vi "11d-async.vi"() -> ()   [LabVIEW 2018, in "LV2Julia_examples.lvlib"]
uses:
  LV2Julia_examples.lvlib
  LV2Julia_core/VIs/Server or client state.ctl
  LV2Julia_core/VIs/detailed error info.ctl
  LV2Julia_core/VIs/StackFrame.ctl
  LV2Julia_core/VIs/Commands.ctl
  be4745b6-8471-45fc-b8a0-8968ce92ea4b.vi
  be4745b6-8471-45fc-b8a0-8968ce92ea4b.vi/01ce1741-ea78-47f8-98ed-e79163fb1a9b.vi
  be4745b6-8471-45fc-b8a0-8968ce92ea4b.vi/01ce1741-ea78-47f8-98ed-e79163fb1a9b.vi/cc3cf2af-bc3b-4fb6-855b-7562c4d0bfeb.vi
  be4745b6-8471-45fc-b8a0-8968ce92ea4b.vi/01ce1741-ea78-47f8-98ed-e79163fb1a9b.vi/c77cecd8-10de-4d46-bc1c-57302a887fda.vi
  be4745b6-8471-45fc-b8a0-8968ce92ea4b.vi/01ce1741-ea78-47f8-98ed-e79163fb1a9b.vi/2cafb1dd-d397-4b79-911a-06d102936120.vi
  LV2Julia_core/VIs/jl-scripts path.vi
  LV2Julia_core/VIs/check ID validity.vi
  LV2Julia_core/VIs/bindata_descr to JSON.vi
  LV2Julia_core/VIs/check cluster field names.vi
  LV2Julia_core/VIs/concat JSON.vi
  LV2Julia_core/VIs/build request.vi
  LV2Julia_core/VIs/Parse server response.vi
  LV2Julia_core/VIs/log jl exceptions.vi
  LV2Julia_core/LV2Julia_core.lvlib
panel:
  in  "Timeout (s)":dbl=-1.0
  out "Boolean":bool
  out "notification":bool
  in  "stop polling":bool
  out "stopping":bool
  out "done":bool
  in  "summands":cluster{"x":dbl, "y":dbl}={"x"=2.0, "y"=2.0}
  in  "next":bool
  out "x+y":dbl=nan
  out "detailed error info":T1
  out "current error":errorcluster
  out "final error":errorcluster
  out "short err code":u8
  in  "stop":bool
  out "ZMQ timeout":bool
  out "Julia script file path":path
  out "temporary script path":path
  out "Jl Server state":T3
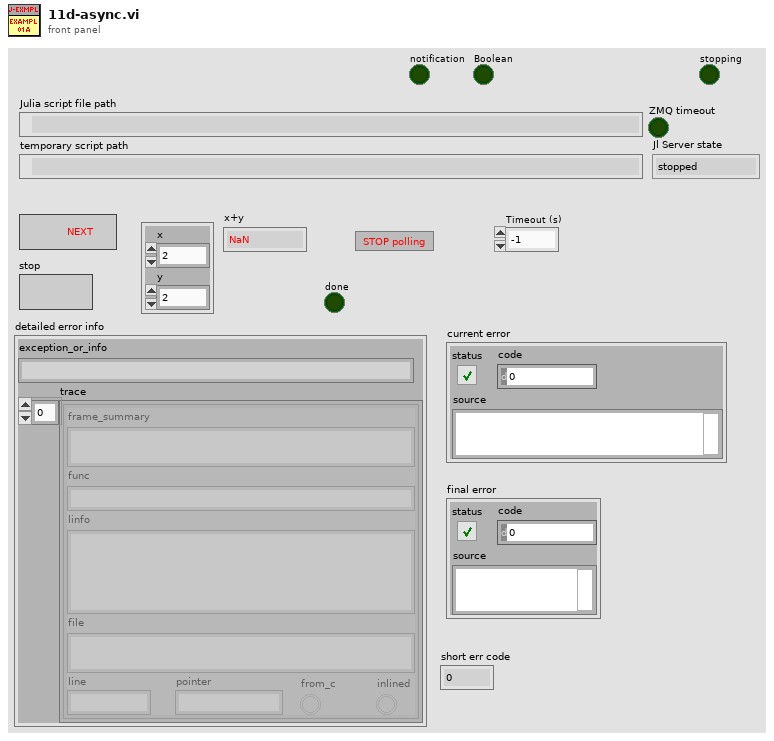
[diagram p1: front panel]
types:
  T1 = typedef "LV2Julia_core.lvlib/detailed error info.ctl" = cluster{"exception_or_info":string, "trace":T2[]}
  T2 = typedef "LV2Julia_core.lvlib/StackFrame.ctl" = cluster{"frame_summary":string, "func":string, "linfo":string, "file":string, "line":i32, "pointer":u64, "from_c":bool, "inlined":bool}
  T3 = typedef "LV2Julia_core.lvlib/Server or client state.ctl" = enum16{"stopped", "running", "unknown"}
  T4 = typedef "LV2Julia_core.lvlib/Commands.ctl" = enum16{"Start Jl-server & Init LV-client", "Send request & Get response ", "Stop Jl-server & Cleanup LV-client", "Cleanup LV-client", "Start Jl-server", "Stop Jl-server", "Init LV-Client", "Cleanup LV-Client", "(not allowed)", "Set LV Client state", "Set Jl Server state", "set ZMQ timeout", "read ZMQ timeout", "read-out state"}
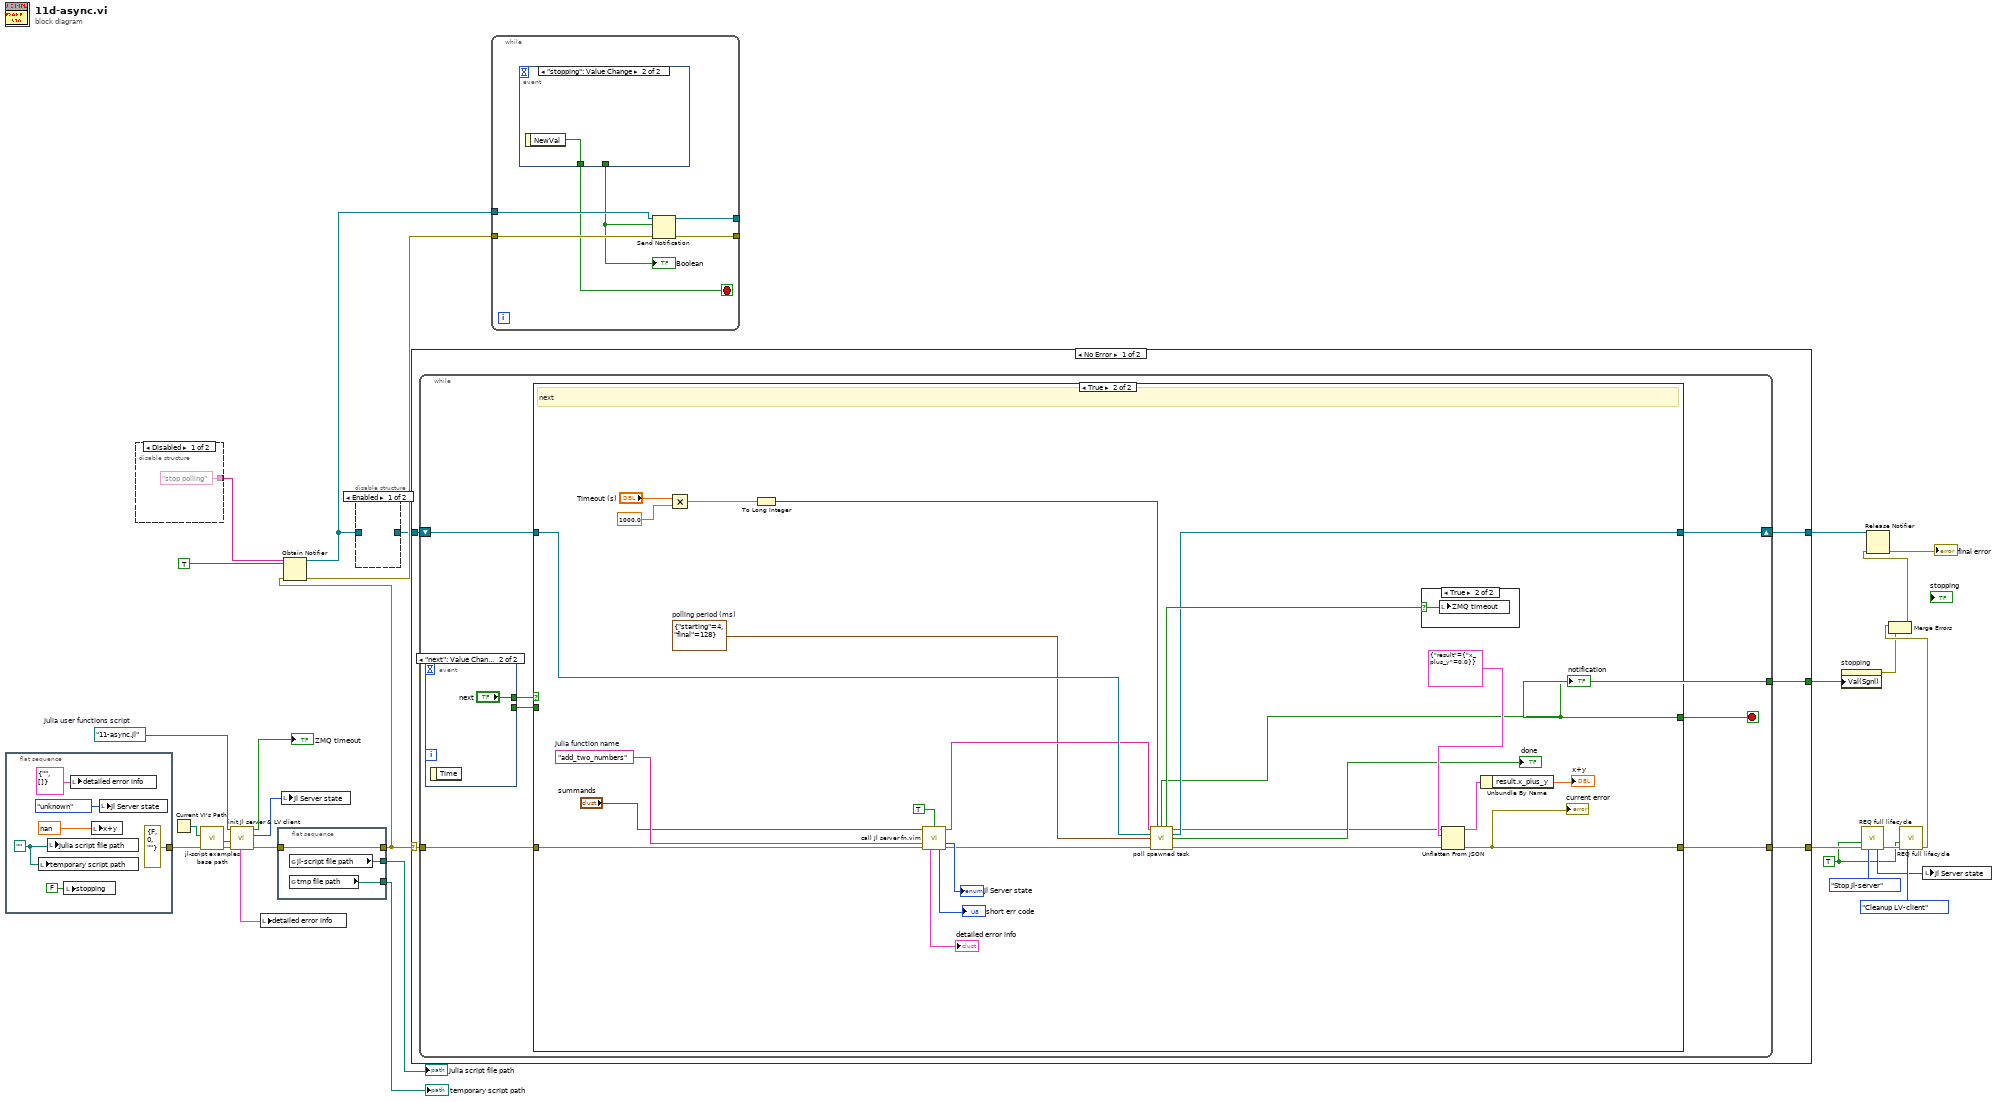
[diagram p0: block diagram]
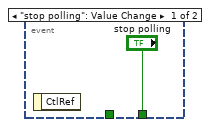
[diagram p4: hidden frame]
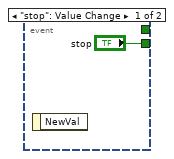
[diagram p5: hidden frame]
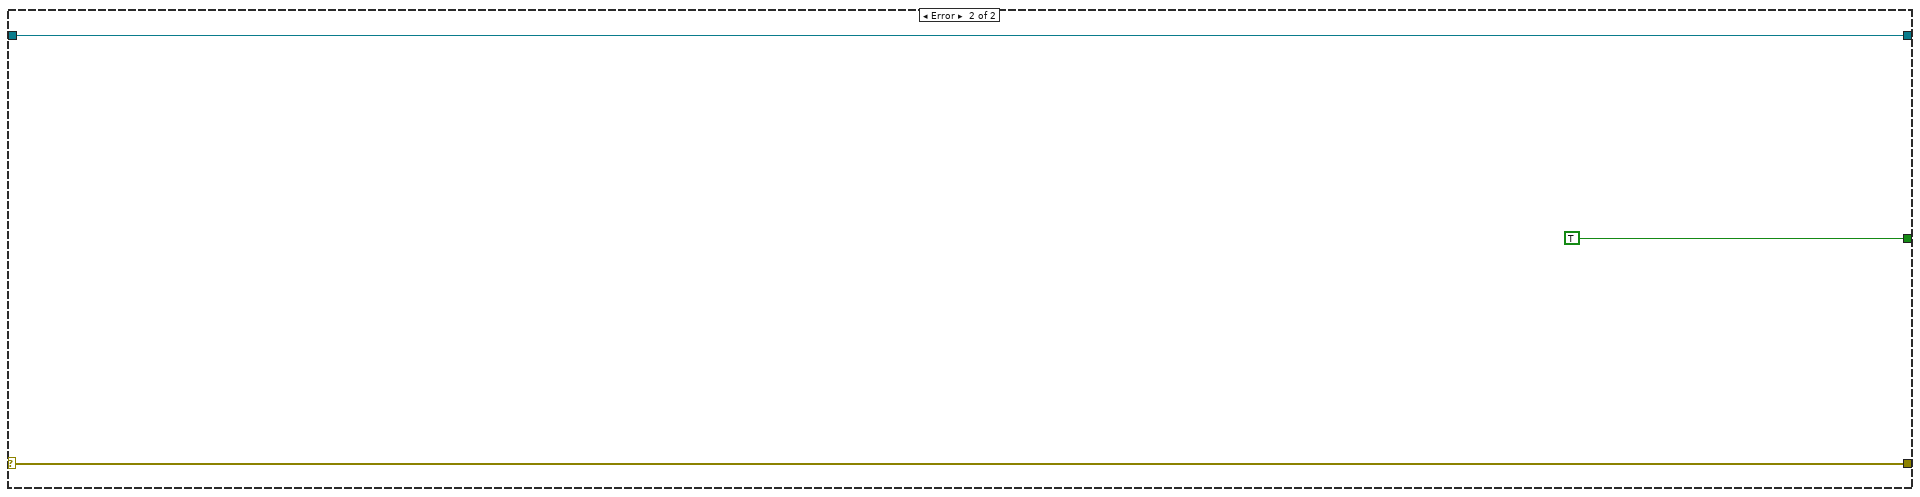
[diagram p8: hidden frame]
diagram:
  w22 = path "11-async.jl"  # Julia user functions script
  w7 = TRUE ("Force command")
  n1 = flat-sequence {
    tunnel: [errorcluster {"status"=FALSE, "code"=0, "source"=""} ("error in (no error)")] -> w18
    frame #0 {
      w31 = path ""
      n2 = local write "temporary script path"(w31) -> ()
      n3 = local write "Julia script file path"(w31) -> ()
      n4 = local write "stopping"(FALSE ("stopping")) -> ()
      n5 = local write "detailed error info"(T1 {"exception_or_info"="", "trace"=[]} ("detailed error info")) -> ()
      n6 = local write "x+y"(nan ("Server response")) -> ()
      n7 = local write "Jl Server state"(Server_or_client_state."unknown" ("Jl Server state out")) -> ()
    }
  }
  n8 = disable-structure shown="Disabled" {
    disable-tunnel: ["stop polling" ("name (unnamed)") _] -> w12
    frame Disabled {
    }
    frame Enabled {
    }
  }
  n9 = Current VI's Path() -> (path=w15:path)
  n10 = call "jl-script examples base path.vi"("error in (no error)"=w18, "calling example VI path"=w15) -> ("error out"=w17:errorcluster, "jl-script-examples base path"=w16:path)  [unwired: 8 in]
  n11 = call "init Jl server & LV client.vi"("error in (no error)"=w17, "Base path (not a path)"=w16, "Julia user functions script"=w22) -> ("error out"=w20:errorcluster, "Jl Server state out"=w19:T3, "timeout?"=→"ZMQ timeout":bool, "detailed error info"=w14:T1)  [unwired: 3 in, 2 out]
  n12 = local write "detailed error info"(w14) -> ()
  n13 = flat-sequence {
    tunnel: [w39] -> w11
    tunnel: w20 -> [w39]
    tunnel: [w38] -> w24
    tunnel: [w37] -> w25
    frame #0 {
      n14 = global read "jl-scripts path.vi" "jl-script file path"() -> (w38:path)
      n15 = global read "jl-scripts path.vi" "tmp file path"() -> (w37:path)
    }
  }
  n16 = local write "Jl Server state"(w19) -> ()
  n17 = Obtain Notifier(name (unnamed)=w12, notification data type=TRUE, error in (no error)=w11) -> (notifier out=w1:refnum<notifier>, error out=w10:errorcluster)  [unwired: 1 in, 1 out]
  n18 = disable-structure shown="Enabled" {
    disable-tunnel: [_ w40] -> w2
    disable-tunnel: w1 -> [_ w40]
    frame Enabled {
    }
    frame Disabled {
    }
  }
  n19 = case shown="No Error" w11 {
    selector: w11 -> [w44 w86]
    tunnel: [w45 w86] -> w29
    tunnel: w2 -> [w43 w85]
    tunnel: [w42 w85] -> w9
    tunnel: [w41 TRUE ("stop")] -> w3
    frame No Error {
      n20 = while {
        tunnel: w44 -> [w51]
        tunnel: [w52] -> w45
        shift-right: [w47] -> w42
        shift-left: w43 -> [w48]
        tunnel: [w46] -> w41
        stop <- w46 stop-if-true
        n21 = event shown="[1] \"next\": Value Change" {
          selector: _ -> [_ _]
          dyn-events: _ -> [_ _]
          timeout: _ -> [_ _]
          tunnel: [_ "next"] -> w50
          tunnel: ["stop" _] -> w49
          event "stop": Value Change {
            n22 = event-data() -> ()  [unwired: 1 in, 1 out]
          }
          event "next": Value Change {
            n23 = event-data() -> ()  [unwired: 1 in, 1 out]
          }
        }
        n24 = case shown="True" w50 {
          tunnel: [w55 w74] -> w52
          tunnel: w51 -> [w55 w76]
          tunnel: [w56 w60] -> w46
          tunnel: w49 -> [w56 _]
          tunnel: w48 -> [w57 w64]
          tunnel: [w57 w62] -> w47
          frame False {
            # "stop"
          }
          frame True {
            w58 = cluster{"starting":i32, "final":i32} {"starting"=4, "final"=128}  # polling period (ms)
            w81 = "add_two_numbers"  # Julia function name
            # "next"
            n25 = Multiply(x="Timeout (s)", y=1000.0) -> (x*y=w67:dbl)
            n26 = To Long Integer(number=w67) -> (32bit integer=w59:i32)
            n27 = call "call Jl server fn.vim"("Arguments 1"="summands", "async call (false)"=TRUE ("timeout?"), "fun2call"=w81, "error in (no error)"=w76) -> ("JSON received"=w63:string, "Jl Server state out"=→"Jl Server state":T3, "detailed error info"=→"detailed error info":T1, "return code"=→"short err code":u8, "error out"=w72:errorcluster)  [unwired: 5 in, 2 out]
            n28 = call "poll spawned task.vi"("JSON string in"=w63, "Timeout, ms (-1)"=w59, "Notifier in"=w64, "polling period (ms)"=w58, "error in (no error)"=w72) -> ("timeout?"=w66:bool, "JSON received"=w61:string, "Notifier out"=w62:refnum<notifier>, "done"=→"done":bool, "Notification out"=w60:bool, "error out"=w71:errorcluster)  [unwired: 2 in, 3 out]
            "notification" <- w60
            n29 = case shown="True" w66 {
              selector: w66 -> [_ w83]
              frame False {
              }
              frame True {
                n30 = local write "ZMQ timeout"(w83) -> ()
              }
            }
            n31 = Unflatten From JSON(JSON string=w61, type and defaults=cluster{"result":cluster{"x_plus_y":dbl}} {"result"={"x_plus_y"=0.0}}, error in (no error)=w71) -> (value=w75:cluster{"result":cluster{"x_plus_y":dbl}}, error out=w74:errorcluster)  [unwired: 4 in]
            "current error" <- w74
            n32 = Unbundle By Name(w75) -> ("result.x_plus_y"=→"x+y":dbl)
          }
        }
      }
    }
    frame Error {
    }
  }
  n33 = while {
    tunnel: w1 -> [w92]
    tunnel: [w91] -> _
    tunnel: w10 -> [w90]
    tunnel: [w89] -> _
    stop <- w87 stop-if-true
    n34 = event shown="[1] \"stopping\": Value Change" {
      selector: _ -> [_ _]
      dyn-events: _ -> [_ _]
      timeout: _ -> [_ _]
      tunnel: ["stop polling" _] -> w88
      tunnel: [_ w94] -> w87
      event "stop polling": Value Change {
        n35 = event-data() -> ()  [unwired: 1 in, 1 out]
      }
      event "stopping": Value Change {
        n36 = event-data() -> ("NewVal"=w94:bool)  [unwired: 1 in]
      }
    }
    "Boolean" <- w88
    n37 = Send Notification(notification=w88, notifier=w92, error in (no error)=w90) -> (notifier out=w91:refnum<notifier>, error out=w89:errorcluster)
  }
  n38 = property on="stopping" class="Bool (strict)"("Val(Sgnl)"=w3) -> (error out=w4:errorcluster)  [unwired: 2 in, 1 out]
  n39 = call "REQ full lifecycle.vi"("Force command"=w7, "error in"=w29, "command"=Commands."Stop Jl-server") -> ("Jl Server state out"=w23:T3, "error out"=w27:errorcluster)  [unwired: 6 in, 5 out]
  n40 = call "REQ full lifecycle.vi"("Force command"=w7, "error in"=w27, "command"=Commands."Cleanup LV-client") -> ("error out"=w6:errorcluster)  [unwired: 6 in, 6 out]
  n41 = Merge Errors(w6, w4) -> (w5:errorcluster)
  n42 = Release Notifier(notifier=w9, error in (no error)=w5) -> (error out=→"final error":errorcluster)  [unwired: 1 in, 2 out]
  n43 = local write "Jl Server state"(w23) -> ()
  "temporary script path" <- w25
  "Julia script file path" <- w24
